vi "LabVIEW-CommEx_Bus_Interface_PWM_SPI_Grad-Buck_v1.3a_Scaled_22Apr2026.vi"() -> ()   [LabVIEW 2018]
uses:
  <vilib>/Instr/_visa.llb/VISA Set IO Buffer Mask.ctl
  <vilib>/Utility/error.llb/DialogType.ctl
  <vilib>/Instr/_visa.llb/VISA Configure Serial Port (Serial Instr).vi
panel:
  out "V_DC_In":dbl format="%.2f"
  out "V_Boost":dbl format="%.2f"
  out "V_Buck":dbl format="%.2f"
  out "V_Pot":dbl format="%.2f"
  in  "LED4_Intensity":dbl(slide)=100.0 scale=0.0..100.0
  in  "LED3_Intensity":dbl(slide)=50.0 scale=0.0..100.0
  in  "LED2_Intensity":dbl(slide)=25.0 scale=0.0..100.0
  in  "LED_BlinkPRD":dbl(slide)=6.2 scale=0.0..100.0
  in  "LED1_Intensity":dbl(slide)=12.5 scale=0.0..100.0
  in  "PWM_En":bool=TRUE
  out "error out 2":errorcluster={"status"=FALSE, "code"=1073676294, "source"="VISA Read in LabVIEW-Int_FPGA_CommExample_2Jun2019_v1.1a_2Jun2019.vi"}
  out "Reg_Array":u16[](array[numeric])=[1, 49151, 24576, 8192, 16384, 32768, 65535, 0, 0, 0, 0, 0, 0, 0, 0, 0, 0, 0, 0, 0, 0, 0, 0, 0, 0, 0, 0, 0, 0, 0, 0, 0, 0, 0, 0, 0, 0, 0, 0, 0, 0, 0, 0, 0, 0, 0, 0, 0, 0, 0, 0, 0, 0, 0, 0, 0, 0, 0, 0, 0, 0, 0, 0, 0] format="%x"
  out "Read_Packet":string
  out "CkSum":bool=TRUE
  out "Recieved Packet":string
  in  "flow control":u16(ring) items=["None"=0, "XON/XOFF"=1, "RTS/CTS"=2, "DTR/DSR"=4]
  in  "Input Buffer Size":u32=16484
  in  "stop 2":bool
  in  "timeout (ms)":u32=100000
  in  "stop bits":u16(ring)=10 items=["1.0"=10, "1.5"=15, "2.0"=20]
  in  "parity":u16(ring) items=["None", "Odd", "Even", "Mark", "Space"]
  in  "data bits":u16=8 min=5 max=8 step=1
  in  "VISA resource name":refnum<visa-resource-name>="COM4"
  in  "baud rate":u32=9600
  out "Cmd_Packet":string
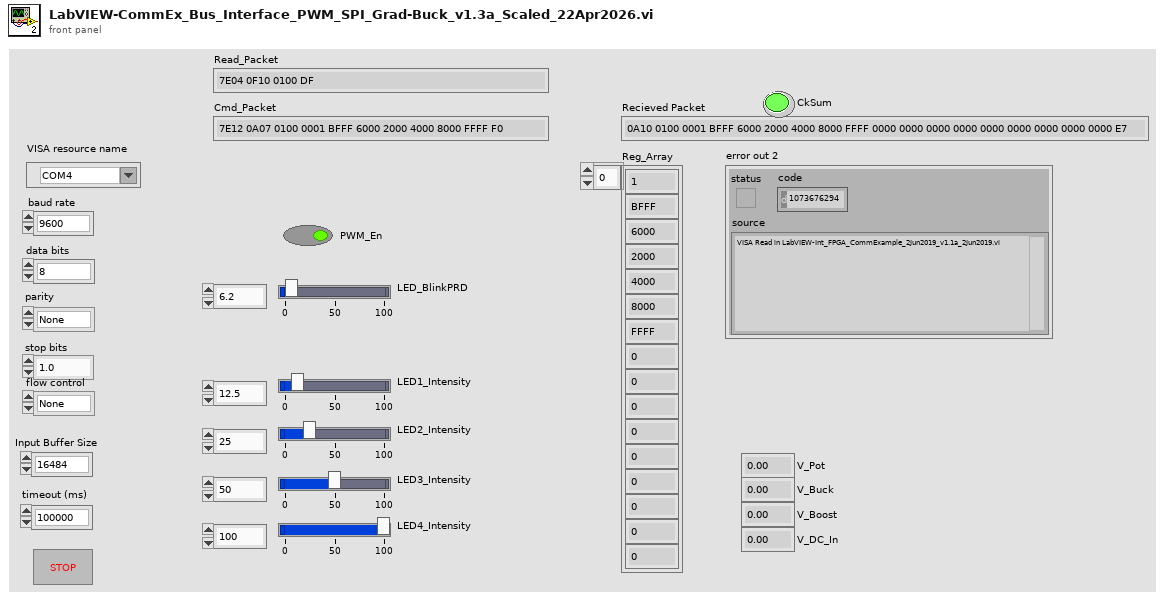
[diagram p1: front panel]
types:
  T1 = typedef "DialogType.ctl" = u16
  T2 = typedef "VISA Set IO Buffer Mask.ctl" = u16
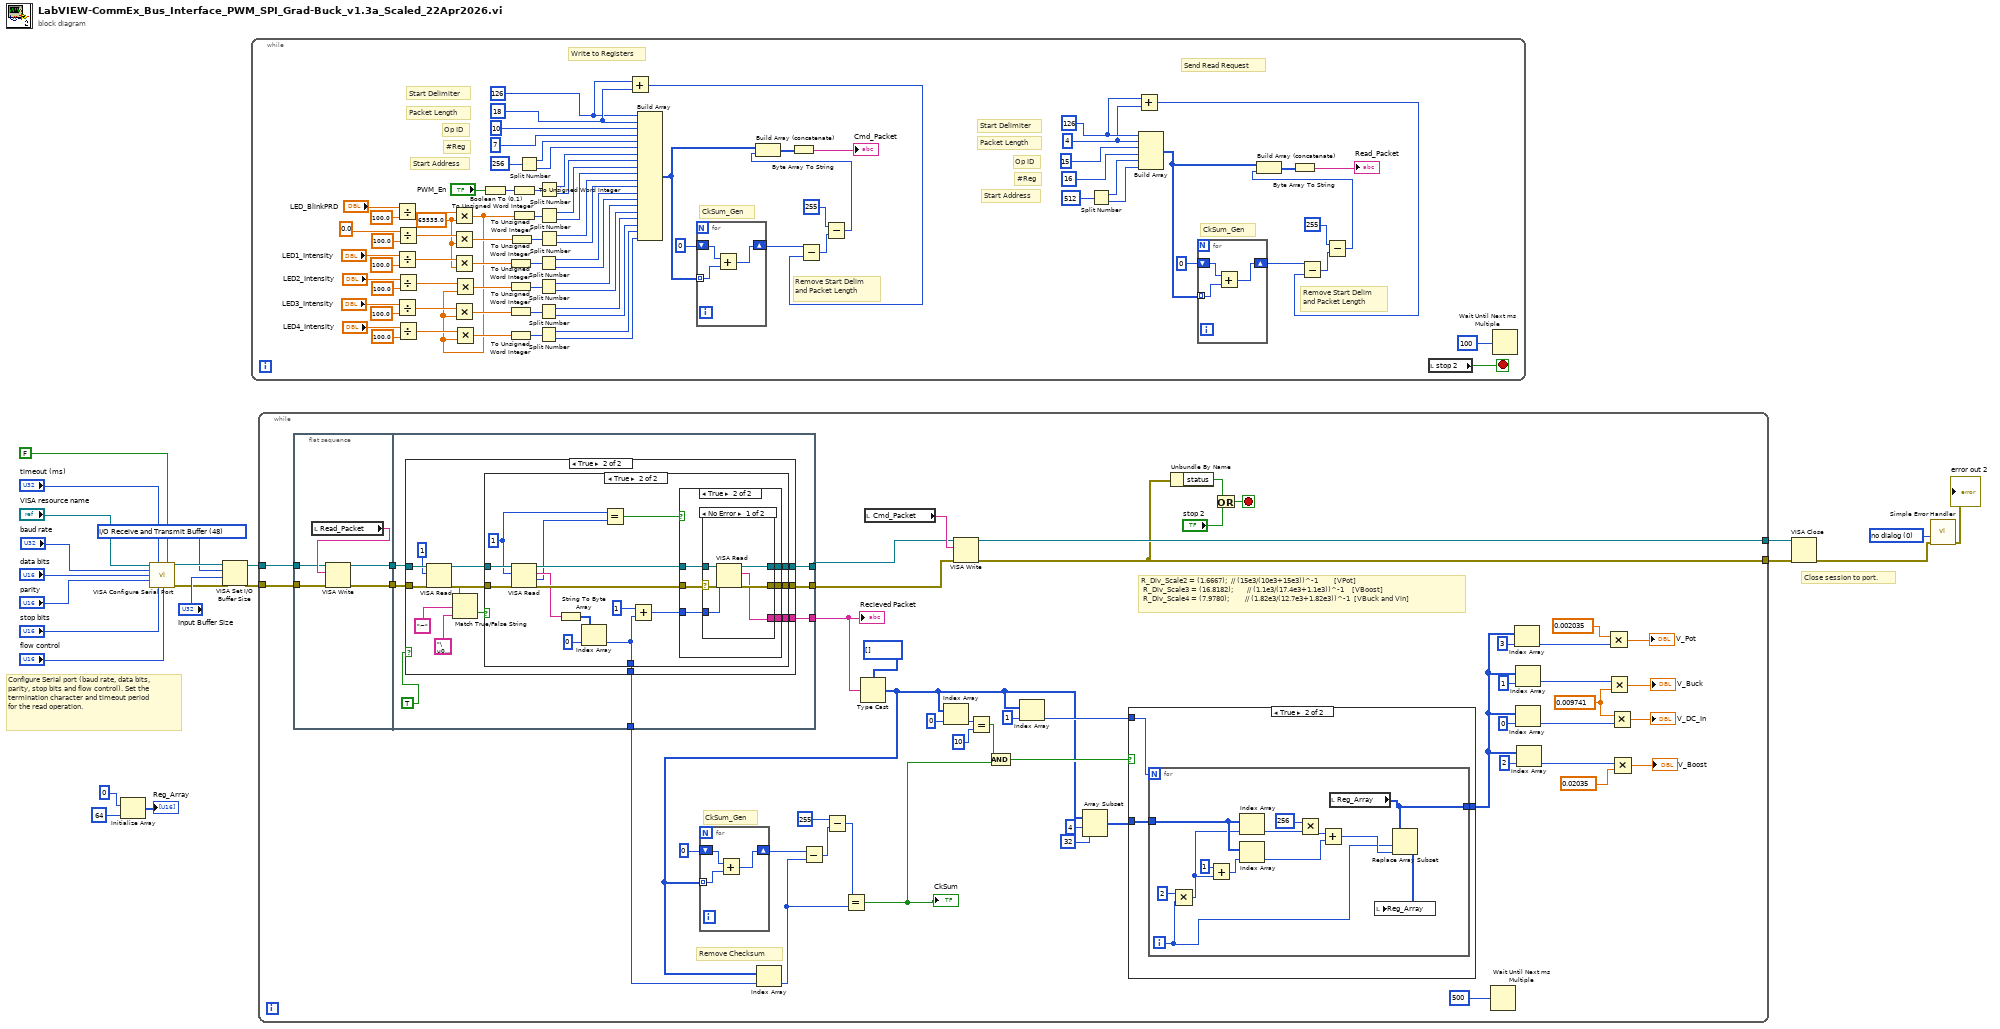
[diagram p0: block diagram]
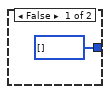
[diagram p2: hidden frame]
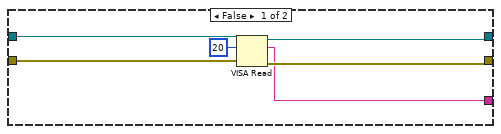
[diagram p3: hidden frame]
diagram:
  w2 = T1 0 items=["no dialog", "OK message", "continue or stop message", "OK message + warnings", "continue/stop + warnings"] ("type of dialog (OK msg:1)")
  w7 = T2 48 items=["I/O Receive Buffer"=16, "I/O Transmit Buffer"=32, "I/O Receive and Transmit Buffer"=48] ("Mask")
  # "Configure Serial port (baud rate, data bits, parity, stop bits and flow control). Set the termination character and timeout period for the read operation."
  # "Close session to port."
  n1 = Initialize Array(u16 0 ("element"), 64 ("dimension size")) -> (→"Reg_Array":u16[])
  n2 = call-poly "VISA Configure Serial Port"("VISA resource name"="VISA resource name", "timeout (10sec)"="timeout (ms)", "Enable Termination\nChar (T)"=FALSE, "baud rate (9600)"="baud rate", "data bits (8)"="data bits", "parity (0:none)"="parity", "stop bits (10: 1 bit)"="stop bits", "flow control (0:none)"="flow control") -> ("VISA resource name out"=w14:refnum<visa-resource-name>, "error out"=w13:errorcluster)  [unwired: 2 in, 4 out]
  n3 = VISA Set I/O Buffer Size(VISA resource name=w14, mask (16)=w7, size (4096)="Input Buffer Size", error in (no error)=w13) -> (VISA resource name out=w10:refnum<visa-resource-name>, error out=w11:errorcluster)
  n4 = while {
    stop <- w94 stop-if-true
    w23 = 65535.0 ("x")
    w27 = u8 4
    w28 = u8 126
    w77 = u8 18
    w76 = u8 126
    # "Write to Registers"
    # "Send Read Request"
    # "#Reg"
    # "Start Address"
    # "Start Delimiter"
    # "Packet Length"
    # "Op ID"
    # "Remove Start Delim\nand Packet Length"
    # "CkSum_Gen"
    # "Remove Start Delim\nand Packet Length"
    # "CkSum_Gen"
    # "#Reg"
    # "Start Address"
    # "Start Delimiter"
    # "Packet Length"
    # "Op ID"
    n5 = Divide(x="LED_BlinkPRD", y=100.0) -> (x/y=w57:dbl)
    n6 = Divide(x="LED1_Intensity", y=100.0) -> (x/y=w52:dbl)
    n7 = Divide(x="LED3_Intensity", y=100.0) -> (x/y=w42:dbl)
    n8 = Divide(x=0.0, y=100.0) -> (x/y=w55:dbl)
    n9 = Divide(x="LED2_Intensity", y=100.0) -> (x/y=w48:dbl)
    n10 = Divide(x="LED4_Intensity", y=100.0) -> (x/y=w38:dbl)
    n11 = Multiply(x=w57, y=w23) -> (x*y=w24:dbl)
    n12 = Multiply(x=w55, y=w23) -> (x*y=w54:dbl)
    n13 = Multiply(x=w52, y=w23) -> (x*y=w51:dbl)
    n14 = Multiply(x=w42, y=w24) -> (x*y=w41:dbl)
    n15 = Multiply(x=w48, y=w24) -> (x*y=w46:dbl)
    n16 = Multiply(x=w38, y=w24) -> (x*y=w36:dbl)
    n17 = Boolean To (0,1)(Boolean="PWM_En") -> (0, 1=w73:i16)
    n18 = To Unsigned Word Integer(number=w51) -> (unsigned 16bit integer=w90:u16)
    n19 = To Unsigned Word Integer(number=w46) -> (unsigned 16bit integer=w89:u16)
    n20 = To Unsigned Word Integer(number=w41) -> (unsigned 16bit integer=w45:u16)
    n21 = To Unsigned Word Integer(number=w36) -> (unsigned 16bit integer=w44:u16)
    n22 = To Unsigned Word Integer(number=w54) -> (unsigned 16bit integer=w91:u16)
    n23 = To Unsigned Word Integer(number=w73) -> (unsigned 16bit integer=w78:u16)
    n24 = To Unsigned Word Integer(number=w24) -> (unsigned 16bit integer=w104:u16)
    n25 = Split Number(x=u16 256) -> (hi(x)=w71:u8, lo(x)=w70:u8)
    n26 = Split Number(x=w90) -> (hi(x)=w63:u8, lo(x)=w62:u8)
    n27 = Split Number(x=w89) -> (hi(x)=w61:u8, lo(x)=w60:u8)
    n28 = Split Number(x=w45) -> (hi(x)=w35:u8, lo(x)=w34:u8)
    n29 = Split Number(x=w44) -> (hi(x)=w33:u8, lo(x)=w32:u8)
    n30 = Split Number(x=w78) -> (hi(x)=w69:u8, lo(x)=w68:u8)
    n31 = Split Number(x=w104) -> (hi(x)=w67:u8, lo(x)=w66:u8)
    n32 = Split Number(x=w91) -> (hi(x)=w65:u8, lo(x)=w64:u8)
    n33 = Add(x=w76, y=w77) -> (x+y=w75:u8)
    n34 = Build Array(w76, w77, u8 10, u8 7, w71, w70, w69, w68, w67, w66, w65, w64, w63, w62, w61, w60, w35, w34, w33, w32) -> (w101:u8[])
    n35 = for {
      tunnel: w101 -> [w108] mode=indexing
      shift-right: [w110] -> w93
      shift-left: u8 0 -> [w109]
      n36 = Add(x=w109, y=w108) -> (x+y=w110:u8)
    }
    n37 = Subtract(x=w93, y=w75) -> (x-y=w92:u8)
    n38 = Subtract(x=u8 255, y=w92) -> (x-y=w95:u8)
    n39 = Build Array (concatenate)(w101, w95) -> (w100:u8[])
    n40 = Byte Array To String(unsigned byte array=w100) -> (string=→"Cmd_Packet":string)
    n41 = Split Number(x=u16 512) -> (hi(x)=w30:u8, lo(x)=w29:u8)
    n42 = Add(x=w28, y=w27) -> (x+y=w26:u8)
    n43 = Build Array(w28, w27, u8 15, u8 16, w30, w29) -> (w87:u8[])
    n44 = for {
      tunnel: w87 -> [w105] mode=indexing
      shift-right: [w107] -> w82
      shift-left: u8 0 -> [w106]
      n45 = Add(x=w106, y=w105) -> (x+y=w107:u8)
    }
    n46 = Subtract(x=w82, y=w26) -> (x-y=w81:u8)
    n47 = Subtract(x=u8 255, y=w81) -> (x-y=w83:u8)
    n48 = Build Array (concatenate)(w87, w83) -> (w86:u8[])
    n49 = Byte Array To String(unsigned byte array=w86) -> (string=→"Read_Packet":string)
    n50 = local read "stop 2"() -> (w94:bool)
    n51 = Wait Until Next ms Multiple(millisecond multiple=u8 100) -> ()  [unwired: 1 out]
  }
  n52 = while {
    tunnel: w11 -> [w144]
    tunnel: w10 -> [w145]
    tunnel: [w149] -> w8
    tunnel: [w132] -> w9
    stop <- w159 stop-if-true
    w118 = 0.009741
    # "R_Div_Scale2 = (1.6667);\t\t// (15e3/(10e3+15e3))^-1        [VPot]\n\tR_Div_Scale3 = (16.8182);       // (1.1e3/(17.4e3+1.1e3))^-1    [VBoost]\n\tR_Div_Scale4 = (7.9780);        // (1.82e3/(12.7e3+1.82e3))^-1  [VBuck and Vin]"
    # "Remove Checksum"
    # "CkSum_Gen"
    n53 = flat-sequence {
      tunnel: [w181] -> w147
      tunnel: [w180] -> w146
      tunnel: w145 -> [w179]
      tunnel: w144 -> [w178]
      tunnel: [w189] -> w148
      tunnel: w147 -> [w188]
      tunnel: w146 -> [w187]
      tunnel: [w186] -> w143
      tunnel: [w185] -> w142
      tunnel: [w183] -> w135
      frame #0 {
        n54 = local read "Read_Packet"() -> (w182:string)
        n55 = VISA Write(VISA resource name=w179, write buffer=w182, error in (no error)=w178) -> (VISA resource name out=w181:refnum<visa-resource-name>, error out=w180:errorcluster)  [unwired: 1 out]
      }
      frame #1 {
        n56 = case shown="True" TRUE {
          tunnel: w187 -> [w194 w205]
          tunnel: w188 -> [w195 w203]
          tunnel: [w192 w208] -> w185
          tunnel: [w193 w207] -> w186
          tunnel: [w190 w206] -> w189
          tunnel: [_ w196] -> w183
          frame False {
            n57 = VISA Read(VISA resource name=w195, byte count=u32 20, error in (no error)=w194) -> (VISA resource name out=w193:refnum<visa-resource-name>, read buffer=w190:string, error out=w192:errorcluster)  [unwired: 1 out]
          }
          frame True {
            n58 = VISA Read(VISA resource name=w203, byte count=u32 1 ("millisecond multiple"), error in (no error)=w205) -> (VISA resource name out=w202:refnum<visa-resource-name>, read buffer=w200:string, error out=w204:errorcluster)  [unwired: 1 out]
            n59 = Match True/False String(2:"\u0000", 3:"~", 4:w200) -> (0:w198:bool)  [unwired: 1 out]
            n60 = case shown="True" w198 {
              tunnel: [w209 w226] -> w208
              tunnel: [w210 w225] -> w207
              tunnel: [_ w224] -> w206
              tunnel: w204 -> [w209 w223]
              tunnel: w202 -> [w210 w222]
              tunnel: [_ w211] -> w196
              frame False {
              }
              frame True {
                w215 = u32 1 ("byte count")
                n61 = VISA Read(VISA resource name=w222, byte count=w215, error in (no error)=w223) -> (VISA resource name out=w221:refnum<visa-resource-name>, read buffer=w218:string, return count=w214:u32, error out=w220:errorcluster)
                n62 = String To Byte Array(string=w218) -> (unsigned byte array=w217:u8[])
                n63 = Index Array(array=w217, index=u32 0 ("millisecond multiple")) -> (element=w211:u8)
                n64 = Equal?(x=w215, y=w214) -> (x = y?=w213:bool)
                n65 = Add(x=u32 1 ("millisecond multiple"), y=w211) -> (x+y=w212:u32)
                n66 = case shown="True" w213 {
                  tunnel: [w227 w234] -> w226
                  tunnel: [w228 w233] -> w225
                  tunnel: w220 -> [w227 w232]
                  tunnel: w221 -> [w228 w231]
                  tunnel: [_ w230] -> w224
                  tunnel: w212 -> [_ w229]
                  frame False {
                  }
                  frame True {
                    n67 = case "Read bytes from port." shown="No Error" w232 {
                      selector: w232 -> [w237 w241]
                      tunnel: [w239 w241] -> w234
                      tunnel: [w240 w242] -> w233
                      tunnel: w231 -> [w238 w242]
                      tunnel: [w235 _] -> w230
                      tunnel: w229 -> [w236 _]
                      frame No Error {
                        n68 = VISA Read(VISA resource name=w238, byte count=w236, error in (no error)=w237) -> (VISA resource name out=w240:refnum<visa-resource-name>, read buffer=w235:string, error out=w239:errorcluster)  [unwired: 1 out]
                      }
                      frame Error {
                        # "Error occurred \nreading Bytes at \nSerial Port"
                      }
                    }
                  }
                }
              }
            }
          }
        }
      }
    }
    n69 = Type Cast(type=u8[] [], x=w148) -> (*(type *) &x=w130:u8[])
    n70 = for {
      tunnel: w130 -> [w243] mode=indexing
      shift-right: [w245] -> w153
      shift-left: u8 0 -> [w244]
      n71 = Add(x=w244, y=w243) -> (x+y=w245:u8)
    }
    n72 = Index Array(array=w130, index=w135) -> (element=w150:u8)
    n73 = Subtract(x=w153, y=w150) -> (x-y=w152:u8)
    n74 = Subtract(x=u8 255, y=w152) -> (x-y=w151:u8)
    n75 = Equal?(x=w151, y=w150) -> (x = y?=w133:bool)
    "CkSum" <- w133
    n76 = local read "Cmd_Packet"() -> (w156:string)
    n77 = Index Array(array=w130, index=0) -> (element=w140:u8)
    n78 = VISA Write(VISA resource name=w143, write buffer=w156, error in (no error)=w142) -> (VISA resource name out=w149:refnum<visa-resource-name>, error out=w132:errorcluster)  [unwired: 1 out]
    n79 = Equal?(x=w140, y=u16 10) -> (x = y?=w138:bool)
    n80 = And(x=w138, y=w133) -> (x .and. y?=w137:bool)
    n81 = Index Array(array=w130, index=1) -> (element=w134:u8)
    n82 = Array Subset(array=w130, index=4, length=32) -> (w129:u8[])
    n83 = case shown="True" w137 {
      tunnel: w134 -> [_ w163]
      tunnel: w129 -> [_ w164]
      tunnel: [u16[] [] ("Reg_Array") w162] -> w114
      frame False {
      }
      frame True {
        n84 = for {
          N: w163 -> [_]
          tunnel: w164 -> [w173]
          tunnel: [w165] -> w162
          i -> [w169]
          n85 = Multiply(x=2, y=w169) -> (x*y=w168:i32)
          n86 = Add(x=1, y=w168) -> (x+y=w166:i32)
          n87 = Index Array(array=w173, index=w168) -> (element=w175:u8)
          n88 = Index Array(array=w173, index=w166) -> (element=w174:u8)
          n89 = Multiply(x=u32 256 ("millisecond multiple"), y=w175) -> (x*y=w177:u32)
          n90 = Add(x=w177, y=w174) -> (x+y=w172:u32)
          n91 = local read "Reg_Array"() -> (w165:u16[])
          n92 = Replace Array Subset(array=w165, new element=w172, index=w169) -> (w171:u16[])
          n93 = local write "Reg_Array"(w171) -> ()
        }
      }
    }
    n94 = Unbundle By Name(w132) -> ("status"=w160:bool)
    n95 = Or(x=w160, y="stop 2") -> (x .or. y?=w159:bool)
    n96 = Wait Until Next ms Multiple(millisecond multiple=u32 500) -> ()  [unwired: 1 out]
    n97 = Index Array(array=w114, index=3) -> (element=w120:u16)
    n98 = Index Array(array=w114, index=0) -> (element=w116:u16)
    n99 = Index Array(array=w114, index=1) -> (element=w117:u16)
    n100 = Index Array(array=w114, index=2) -> (element=w115:u16)
    n101 = Multiply(x=0.002035, y=w120) -> (x*y=→"V_Pot":dbl)
    n102 = Multiply(x=w117, y=w118) -> (x*y=→"V_Buck":dbl)
    n103 = Multiply(x=w118, y=w116) -> (x*y=→"V_DC_In":dbl)
    n104 = Multiply(x=w115, y=0.02035) -> (x*y=→"V_Boost":dbl)
    "Recieved Packet" <- w148
  }
  n105 = VISA Close(VISA resource name=w8, error in (no error)=w9) -> (error out=w1:errorcluster)
  n106 = call <vilib>:"Simple Error Handler.vi"("type of dialog (OK msg:1)"=w2, "error in (no error)"=w1) -> ("error out"=→"error out 2":errorcluster)  [unwired: 7 out]
